vi "build.from.objects.vi"(11 "volume objects":cluster{"Array":T2[]}[](array[cluster])) -> (2 "Report":T1[](array[typedef]) {"cover_date" format="%<%x>T"}, 3 "Exported Report":string[][](array[string]))   [LabVIEW 2024]
uses:
  graphics/volume.object--cluster.ctl
  definitions/volume.type--enum.ctl
  comic_manager/TypeDefs/issue.display--cluster.ctl
  report.issue--cluster.ctl
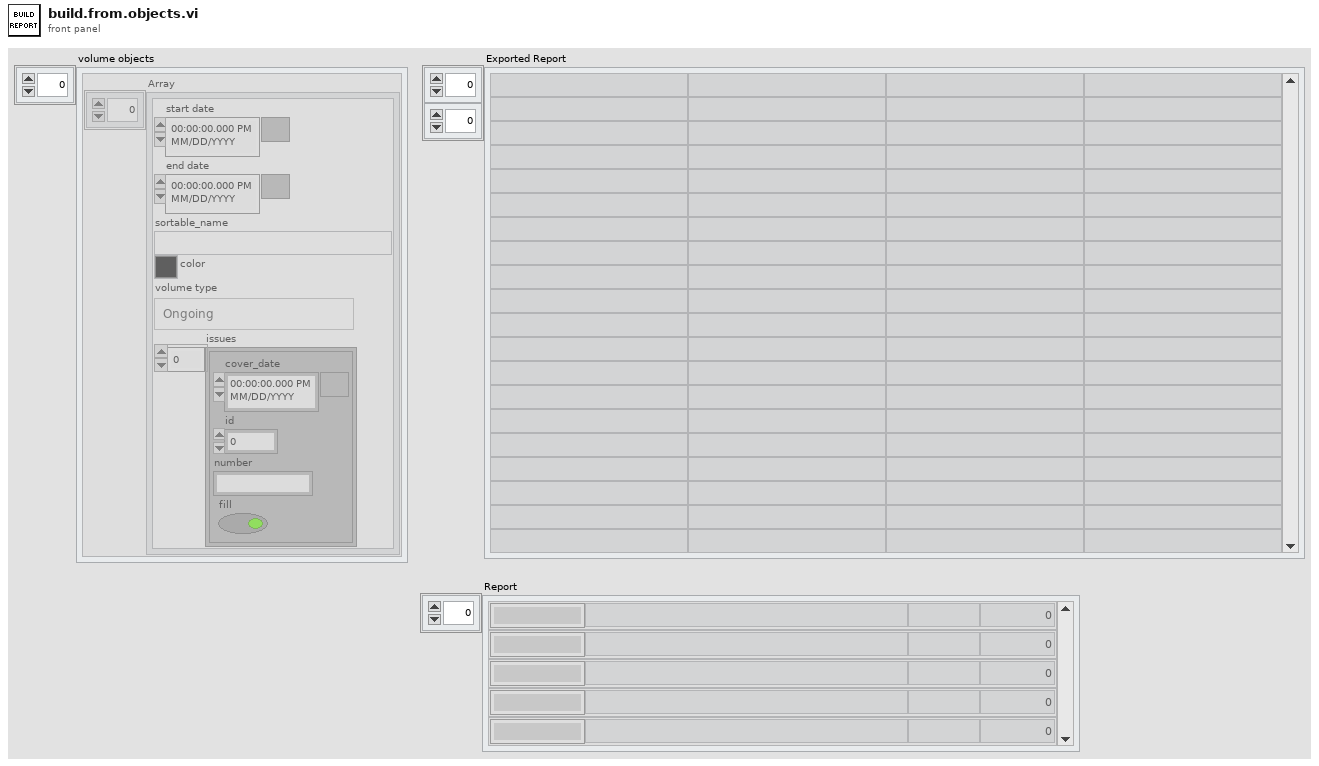
[diagram p1: front panel]
types:
  T1 = typedef "report.issue--cluster.ctl" = cluster{"cover_date":timestamp, "sortable_name":string, "number":string, "id":i32}
  T2 = typedef "volume.object--cluster.ctl" = cluster{"start date":timestamp, "end date":timestamp, "sortable_name":string, "color":u32, "volume type":T3, "issues":T4[]}
  T3 = typedef "volume.type--enum.ctl" = enum16{"Ongoing", "Limited Series", "Annual", "One Shot", "Reprint/Document", "Star Comics", "Epic Comics"}
  T4 = typedef "issue.display--cluster.ctl" = cluster{"cover_date":timestamp, "id":i32, "number":string, "fill":bool}
  T5 = cluster{"cover_date":timestamp, "result string":string, "number":string, "id":i32}
  T6 = cluster{"cover_date":timestamp, "result string":string, "number":string, "id":i32}[]
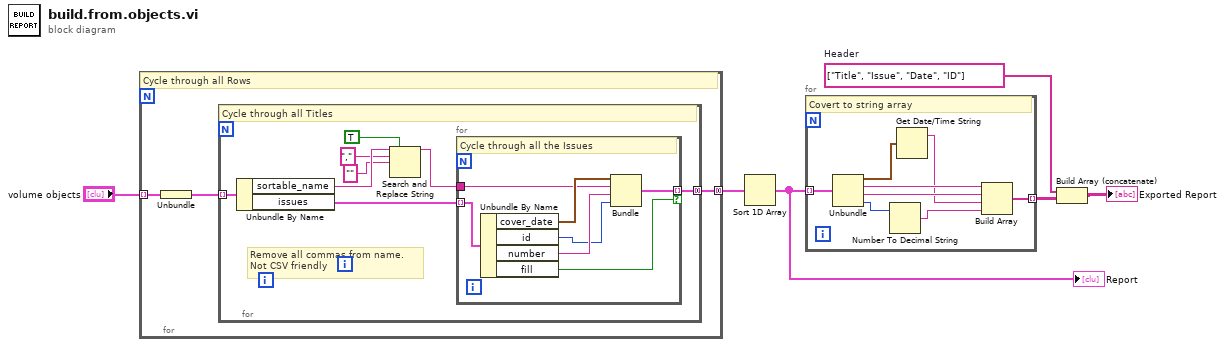
[diagram p0: block diagram]
diagram:
  w3 = string[] ["Title", "Issue", "Date", "ID"]  # Header
  n1 = for {
    tunnel: "volume objects" -> [w9] mode=indexing
    tunnel: [w7] -> w5 mode=concatenating
    # "Cycle through all Rows"
    n2 = Unbundle(w9) -> ("Array"=w8:T2[])
    n3 = for {
      tunnel: w8 -> [w17] mode=indexing
      tunnel: [w15] -> w7 mode=concatenating
      # "Remove all commas from name.\nNot CSV friendly"
      # "Cycle through all Titles"
      n4 = Unbundle By Name(w17) -> ("sortable_name"=w14:string, "issues"=w16:T4[])
      n5 = Search and Replace String(replace all?=TRUE ("replace all? (F)"), input string=w14, search string=",", replace string="" ("replace string (\"\")")) -> (result string=w10:string)  [unwired: 4 in, 3 out]
      n6 = for {
        tunnel: w16 -> [w24] mode=indexing
        tunnel: w10 -> [w22]
        tunnel: [w19] -> w15 mode=indexing if=w18
        # "Cycle through all the Issues"
        n7 = Unbundle By Name(w24) -> ("cover_date"=w23:timestamp, "id"=w20:i32, "number"=w21:string, "fill"=w18:bool)
        n8 = Bundle("cover_date"=w23, "result string"=w22, "number"=w21, "id"=w20) -> (w19:T5)  [unwired: 1 in]
      }
    }
  }
  n9 = Sort 1D Array(array=w5) -> (sorted array=w1:T6)
  "Report" <- w1
  n10 = for {
    tunnel: w1 -> [w32] mode=indexing
    tunnel: [w25] -> w4 mode=indexing
    # "Covert to string array"
    n11 = Unbundle(w32) -> ("cover_date"=w31:timestamp, "result string"=w30:string, "number"=w29:string, "id"=w28:i32)
    n12 = Number To Decimal String(number=w28) -> (decimal integer string=w27:string)  [unwired: 1 in]
    n13 = Get Date/Time String(seconds (now)=w31) -> (date string=w26:string)  [unwired: 2 in, 1 out]
    n14 = Build Array(w30, w29, w26, w27) -> (w25:string[])
  }
  n15 = Build Array (concatenate)(w3, w4) -> (→"Exported Report":string[][])
